vi "BRig_Host__Loop_Producer__tcp_System__Data.vi"(0 "input_strCmd":string) -> ()   [LabVIEW 2014]
uses:
  myRIO_BRig_RT__Case_Exp_stateList.ctl
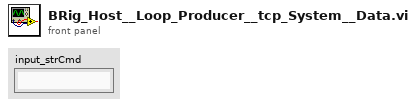
[diagram p1: front panel]
types:
  T1 = typedef "myRIO_BRig_RT__Case_Exp_stateList.ctl" = enum16{"Start1", "Start2", "Start3", "saveSettings1", "saveSettings2", "saveSettings3", "saveSettings4", "saveSettings_LC_ENL_l1", "saveSettings_LC_ENL_l2", "saveSettings_LC_Cue_l1", "saveSettings_LC_Cue_l2", "saveSettings6_LC_l1_Other", "SaveSettings6_LC_l2_Other", "setSettings_Audio", "setSettings_Laser", "initBlock_pre", "initBlock", "initBlock2", "initBlock_post", "initTrial_pre", "initTrial", "initTrial2", "initTrial3", "initTrial4", "initTrial_LC_ENL1", "initTrial_LC_Cue1", "initTrial_LC_Cue1_2", "initTrial_LC_Sel", "initTrial_post", "ENL1_pre", "ENL1", "ENL1_post", "ENL1Penalty_pre", "ENL1Penalty", "ENL2_pre", "ENL2", "ENL2Penalty_pre", "ENL2Penalty", "Cue1_pre", "Cue1", "Cue1_post", "Cue1Penalty_pre", "Cue1Penalty", "Cue2_pre", "Cue2", "Cue2Penalty_pre", "Cue2Penalty", "Selection_pre", "Selection", "Select_post", "SelectReward_pre", "SelectReward", "SelectRewardPost_pre", "SelectRewardPost", "SelectWrong_pre", "SelectWrong", "SelectWrong_post", "SelectTimeout_pre", "SelectTimeout", "SelectTimeout_post", "endTrial_pre", "endTrial1", "endTrial2", "endTrial3", "endTrial_post", "endBlock_pre", "endBlock", "endBlock_post", "endExp", "commConnect", "commUpload_pre", "commUpload_dataBlock", "commUpload_dataCurrent", "commUpload_dataExp", "commUpload_dataLC", "commUpload_dataTrial", "commUpload_post", "saveData_pre", "saveData_dataBlock", "saveData_dataCurrent", "saveData_dataExp", "saveData_dataLC", "saveData_dataTrial", "saveData_post", "empty_endBlock1", "empty_endBlock2", "empty_endTrial1", "empty_endTrial2", "empty_endTrial3", "empty_endTrial4", "empty_endTrial5", "dummyState", "dummyState_endBlock", "FreeReward_pre", "FreeReward", "FreeRewardPost_pre", "FreeRewardPost"}
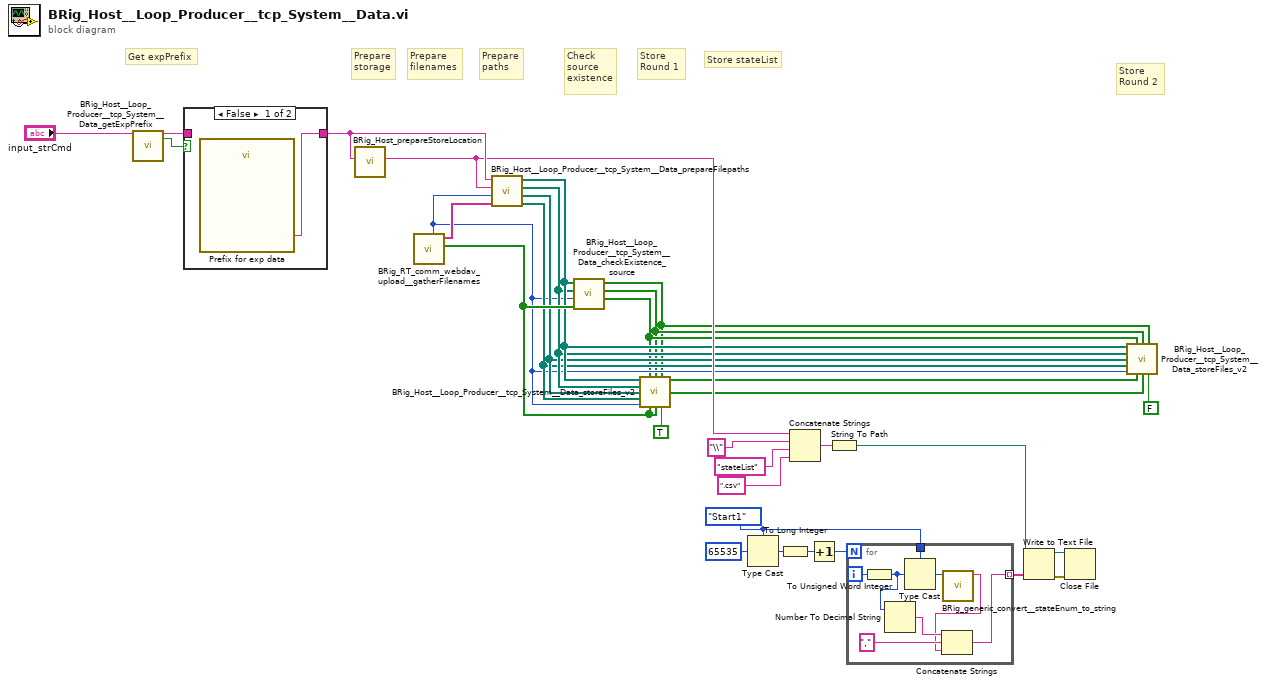
[diagram p0: block diagram]
diagram:
  w17 = myRIO_BRig_RT__Case_Exp_stateList."Start1" ("Enum")
  # "Store\nRound 2"
  # "Store stateList"
  # "Store\nRound 1"
  # "Check\nsource\nexistence"
  # "Prepare\npaths"
  # "Prepare\nfilenames"
  # "Prepare\nstorage"
  # "Get expPrefix"
  n1 = call "BRig_Host__Loop_Producer__tcp_System__Data_getExpPrefix.vi"("input_strCmd"="input_strCmd") -> ("output_expPrefix"=w30:string, "output_I_expPrefix"=w31:bool)  [unwired: 17 in]
  n2 = case shown="False" w31 {
    tunnel: w30 -> [_ w34]
    tunnel: [w33 w34] -> w29
    frame False {
      n3 = call "Prefix for exp data"() -> ("expPrefix"=w33:string)  [unwired: 17 in, 2 out]
    }
    frame True {
    }
  }
  n4 = call "BRig_Host_prepareStoreLocation.vi"("input_expPrefix"=w29) -> ("output_folderPath"=w26:string)  [unwired: 9 in, 1 out]
  n5 = call "BRig_RT_comm_webdav_upload__gatherFilenames.vi"() -> ("output_arrBlank"=w27:bool[], "output_arrFilenames"=w28:string[], "output_n"=w7:i32)  [unwired: 9 in]
  n6 = call "BRig_Host__Loop_Producer__tcp_System__Data_prepareFilepaths.vi"("input_arrFilenames"=w28, "input_nFilenames"=w7, "input_storagePath"=w26, "input_expPrefix"=w29) -> ("output_arrPath_target"=w8:path[], "output_arrPath_target_wExpPrefix"=w9:path[], "output_arrPath_source"=w10:path[], "output_arrPath_source_wExpPrefix"=w11:path[])  [unwired: 4 in]
  n7 = call "BRig_Host__Loop_Producer__tcp_System__Data_checkExistence_source.vi"("input_I_arrPath"=w27, "input_n"=w7, "input_arrPath_source"=w10, "input_arrPath_source_wExpPrefix"=w11) -> ("output_exist_sourceAny"=w4:bool[], "output_exist_source"=w3:bool[], "output_exist_source_wExpPrefix"=w2:bool[])  [unwired: 5 in]
  n8 = call "BRig_Host__Loop_Producer__tcp_System__Data_storeFiles_v2.vi"("input_arrPath_source_wExpPrefix"=w11, "input_exist_sourceAny"=w4, "input_exist_source"=w3, "input_exist_source_wExpPrefix"=w2, "input_arrPath_source"=w10, "input_arrPath_target_wExpPrefix"=w9, "input_arrPath_target"=w8, "input_n"=w7, "input_store_wExpPrefix"=w27, "input_storeAny"=w27, "input_firstPass"=TRUE) -> ("output_stored_wExpPrefix"=w6:bool[], "output_storedAny"=w5:bool[])  [unwired: 3 in]
  n9 = Type Cast(type=w17, x=u16 65535) -> (*(type *) &x=w20:T1)
  n10 = To Long Integer(number=w20) -> (32bit integer=w19:i32)
  n11 = Concatenate Strings(w26, "\\" ("string"), "stateList" ("input_fileName"), ".csv" ("string")) -> (w22:string)
  n12 = Increment(x=w19) -> (x+1=w18:i32)
  n13 = String To Path(string=w22) -> (path=w15:path)
  n14 = for {
    N: w18 -> [_]
    tunnel: w17 -> [w41]
    tunnel: [w35] -> w16 mode=indexing
    i -> [w40]
    n15 = To Unsigned Word Integer(number=w40) -> (unsigned 16bit integer=w37:u16)
    n16 = Number To Decimal String(number=w37) -> (decimal integer string=w38:string)  [unwired: 1 in]
    n17 = Type Cast(type=w41, x=w37) -> (*(type *) &x=w42:T1)
    n18 = call "BRig_generic_convert__stateEnum_to_string.vi"("input_stateEnum"=w42) -> ("output_str"=w36:string)  [unwired: 10 in]
    n19 = Concatenate Strings(w38, ",", w36) -> (w35:string)
  }
  n20 = Write to Text File(file (use dialog)=w15, text=w16) -> (refnum out=w14:refnum<file>, error out=w13:errorcluster)  [unwired: 2 in, 1 out]
  n21 = Close File(refnum=w14, error in=w13) -> ()  [unwired: 2 out]
  n22 = call "BRig_Host__Loop_Producer__tcp_System__Data_storeFiles_v2.vi"("input_arrPath_source_wExpPrefix"=w11, "input_exist_sourceAny"=w4, "input_exist_source"=w3, "input_exist_source_wExpPrefix"=w2, "input_arrPath_source"=w10, "input_arrPath_target_wExpPrefix"=w9, "input_arrPath_target"=w8, "input_n"=w7, "input_store_wExpPrefix"=w6, "input_storeAny"=w5, "input_firstPass"=FALSE) -> ()  [unwired: 3 in, 2 out]
